vi "rmad logger initfile.vi"(0 "initfile":string="rmad config.ini", 11 "error in (no error)":errorcluster) -> (1 "mesh_datadir":string, 2 "aux_datadir":string, 3 "event_datadir":string, 4 "serial mux":T2={"serial_mux IP"="127.0.0.1", "rserial_mux port"=9900}, 6 "RMAD signalys monitor enabled":bool, 7 "ini file":path, 8 "num nodes":u32, 9 "vdv_datadir":string, 10 "num sensors":u32[](array[numeric]), 12 "gateway_snmp":bool, 13 "auto_download":bool, 14 "mac adresses":T1, 15 "error out":errorcluster)   [LabVIEW 2017]
uses:
  <vilib>/Utility/config.llb/Read Key (String).vi
  <vilib>/Utility/config.llb/Read Key (U32).vi
  <vilib>/Utility/config.llb/Read Key (Boolean).vi
  <vilib>/Utility/config.llb/NI_LVConfig.lvlib
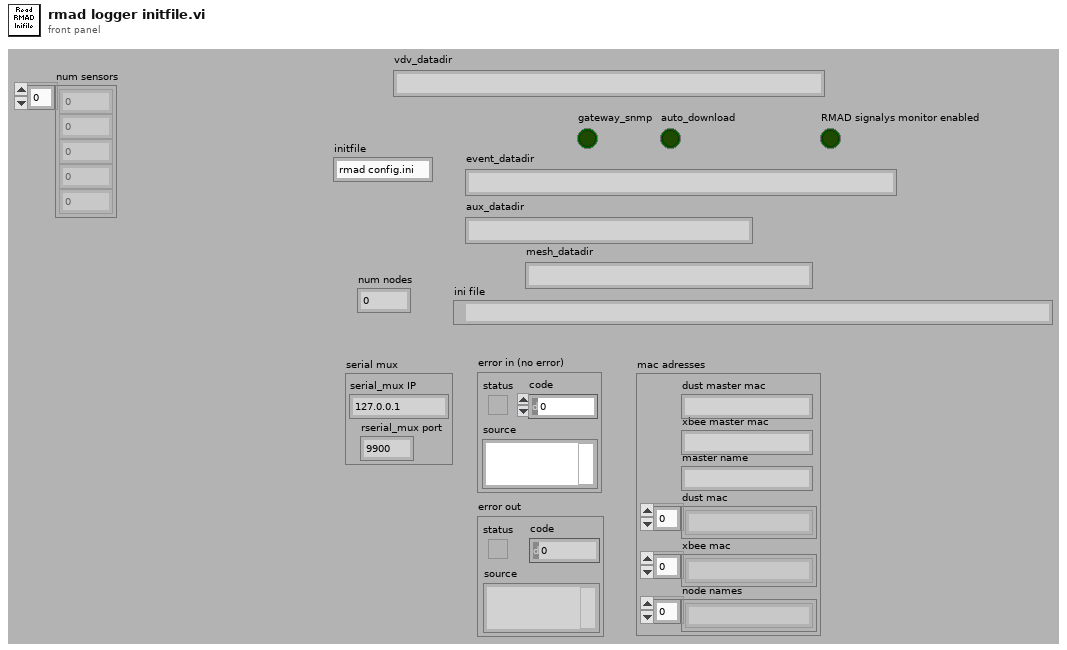
[diagram p1: front panel]
types:
  T1 = cluster{"dust master mac":string, "xbee master mac":string, "master name":string, "dust mac":string[], "xbee mac":string[], "node names":string[]}
  T2 = cluster{"serial_mux IP":string, "rserial_mux port":u16}
  T3 = typedef "NI_LVConfig.lvlib/Config Data RefNum.ctl" = refnum<k1>
  T4 = cluster{"section":string, "section":string, "section":string, string[], string[], string[]}
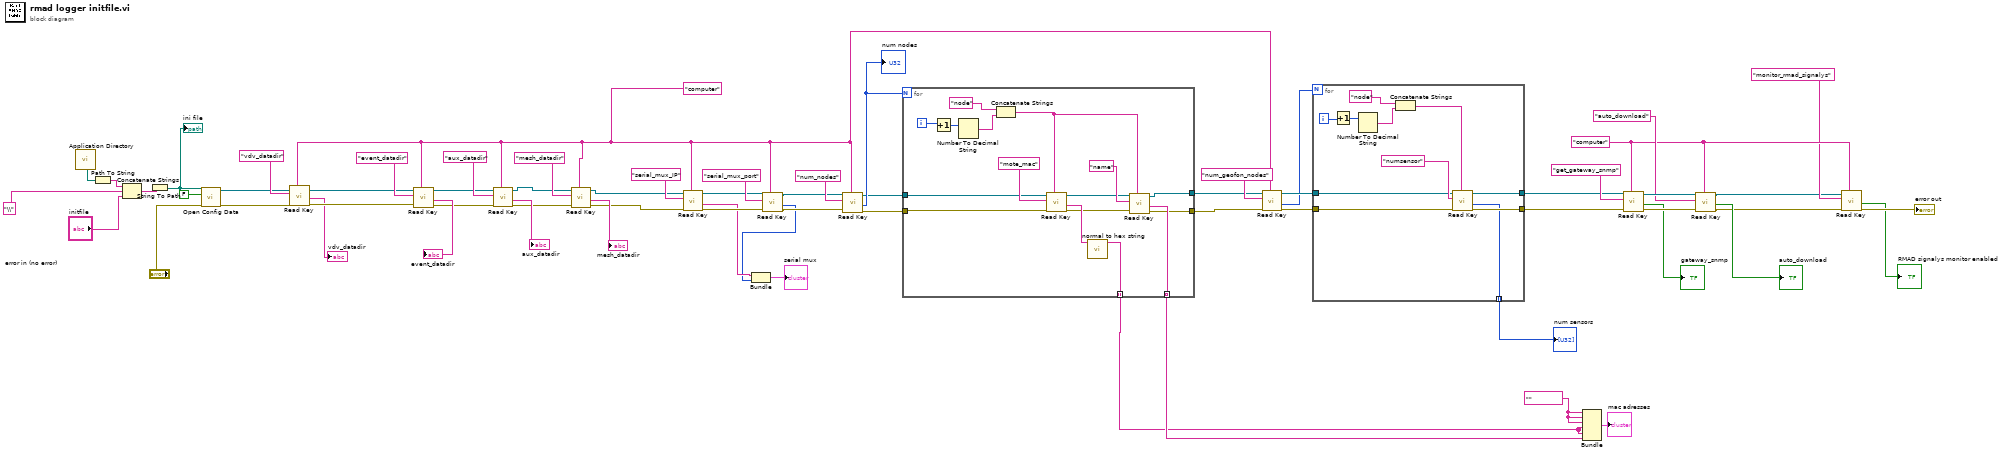
[diagram p0: block diagram]
diagram:
  w11 = "" ("section")
  w23 = "computer" ("section")
  w7 = "computer" ("section")
  n1 = call <vilib>:"Application Directory.vi"() -> ("Application Directory"=w65:path)
  n2 = Path To String(path=w65) -> (string=w64:string)
  n3 = Concatenate Strings(w64, "\\", "initfile") -> (w62:string)
  n4 = String To Path(string=w62) -> (path=w61:path)
  "ini file" <- w61
  n5 = call <vilib>:"Open Config Data.vi"("error in (no error)"="error in (no error)", "create file if necessary (T)"=FALSE, "configuration file path"=w61) -> ("error out"=w19:errorcluster, "refnum"=w18:T3)  [unwired: 6 in, 1 out]
  n6 = call-poly <vilib>:"Read Key.vi"("section"=w7, "error in (no error)"=w19, "key"="vdv_datadir", "refnum"=w18) -> ("error out"=w17:errorcluster, "value"=→"vdv_datadir":string, "refnum out"=w16:T3)  [unwired: 4 in, 1 out]
  n7 = call-poly <vilib>:"Read Key.vi"("section"=w7, "error in (no error)"=w17, "key"="event_datadir", "refnum"=w16) -> ("error out"=w36:errorcluster, "value"=→"event_datadir":string, "refnum out"=w35:T3)  [unwired: 4 in, 1 out]
  n8 = call-poly <vilib>:"Read Key.vi"("section"=w7, "error in (no error)"=w36, "key"="aux_datadir", "refnum"=w35) -> ("error out"=w33:errorcluster, "value"=→"aux_datadir":string, "refnum out"=w34:T3)  [unwired: 4 in, 1 out]
  n9 = call-poly <vilib>:"Read Key.vi"("section"=w7, "error in (no error)"=w33, "key"="mesh_datadir", "refnum"=w34) -> ("error out"=w31:errorcluster, "value"=→"mesh_datadir":string, "refnum out"=w32:T3)  [unwired: 4 in, 1 out]
  n10 = call-poly <vilib>:"Read Key.vi"("section"=w7, "error in (no error)"=w31, "key"="serial_mux_IP", "refnum"=w32) -> ("error out"=w54:errorcluster, "value"=w50:string, "refnum out"=w55:T3)  [unwired: 4 in, 1 out]
  n11 = call-poly <vilib>:"Read Key.vi"("section"=w7, "error in (no error)"=w54, "key"="serial_mux_port", "refnum"=w55) -> ("error out"=w52:errorcluster, "value"=w49:u32, "refnum out"=w53:T3)  [unwired: 4 in, 1 out]
  n12 = Bundle("value"=w50, "value"=w49) -> (→"serial mux":cluster{"value":string, "value":u32})  [unwired: 1 in]
  n13 = call-poly <vilib>:"Read Key.vi"("section"=w7, "error in (no error)"=w52, "key"="num_nodes", "refnum"=w53) -> ("error out"=w47:errorcluster, "value"=w48:u32, "refnum out"=w46:T3)  [unwired: 4 in, 1 out]
  "num nodes" <- w48
  n14 = for {
    N: w48 -> [_]
    tunnel: [w74] -> w43 mode=indexing
    tunnel: w47 -> [w71]
    tunnel: w46 -> [w72]
    tunnel: [w73] -> w44 mode=indexing
    tunnel: [w67] -> w9
    tunnel: [w66] -> w8
    i -> [w78]
    n15 = Increment(x=w78) -> (x+1=w77:i32)
    n16 = Number To Decimal String(number=w77) -> (decimal integer string=w79:string)  [unwired: 1 in]
    n17 = Concatenate Strings("node" ("string"), w79) -> (w68:string)
    n18 = call-poly <vilib>:"Read Key.vi"("section"=w68, "error in (no error)"=w71, "key"="mote_mac" ("section"), "refnum"=w72) -> ("error out"=w70:errorcluster, "value"=w75:string, "refnum out"=w69:T3)  [unwired: 4 in, 1 out]
    n19 = call "normal to hex string.vi"("Normal String"=w75) -> ("Hex Display Sting"=w74:string)  [unwired: 10 in]
    n20 = call-poly <vilib>:"Read Key.vi"("section"=w68, "error in (no error)"=w70, "key"="name", "refnum"=w69) -> ("error out"=w66:errorcluster, "value"=w73:string, "refnum out"=w67:T3)  [unwired: 4 in, 1 out]
  }
  n21 = call-poly <vilib>:"Read Key.vi"("section"=w7, "error in (no error)"=w8, "key"="num_geofon_nodes", "refnum"=w9) -> ("error out"=w6:errorcluster, "value"=w4:u32, "refnum out"=w5:T3)  [unwired: 4 in, 1 out]
  n22 = for {
    N: w4 -> [_]
    tunnel: w6 -> [w85]
    tunnel: w5 -> [w86]
    tunnel: [w84] -> w3
    tunnel: [w83] -> w2
    tunnel: [w82] -> w1 mode=indexing
    i -> [w88]
    n23 = Increment(x=w88) -> (x+1=w89:i32)
    n24 = Number To Decimal String(number=w89) -> (decimal integer string=w90:string)  [unwired: 1 in]
    n25 = Concatenate Strings("node" ("string"), w90) -> (w87:string)
    n26 = call-poly <vilib>:"Read Key.vi"("section"=w87, "error in (no error)"=w85, "key"="numsensor", "refnum"=w86) -> ("error out"=w83:errorcluster, "value"=w82:u32, "refnum out"=w84:T3)  [unwired: 4 in, 1 out]
  }
  "num sensors" <- w1
  n27 = Bundle("section"=w11, "section"=w11, "section"=w11, w43, w43, w44) -> (→"mac adresses":T4)  [unwired: 1 in]
  n28 = call-poly <vilib>:"Read Key.vi"("section"=w23, "error in (no error)"=w2, "key"="get_gateway_snmp", "refnum"=w3) -> ("error out"=w30:errorcluster, "value"=→"gateway_snmp":bool, "refnum out"=w29:T3)  [unwired: 4 in, 1 out]
  n29 = call-poly <vilib>:"Read Key.vi"("section"=w23, "error in (no error)"=w30, "key"="auto_download", "refnum"=w29) -> ("error out"=w12:errorcluster, "value"=→"auto_download":bool, "refnum out"=w13:T3)  [unwired: 4 in, 1 out]
  n30 = call-poly <vilib>:"Read Key.vi"("section"=w23, "error in (no error)"=w12, "key"="monitor_rmad_signalys", "refnum"=w13) -> ("error out"=→"error out":errorcluster, "value"=→"RMAD signalys monitor enabled":bool)  [unwired: 4 in, 2 out]
